vi "Double to Bool.vi"(3 "Double":dbl) -> (1 "Bool":bool)   [LabVIEW 2020, in "Vecto.lvlib"]
uses:
  Vecto.lvlib
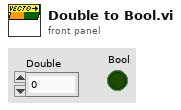
[diagram p1: front panel]
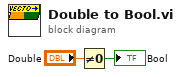
[diagram p0: block diagram]
diagram:
  n1 = Not Equal To 0?(x="Double") -> (x != 0?=→"Bool":bool)
